vi "Indent.vi"(0 "string in":string, 1 "start indentation":i32=1) -> (2 "string out":string)   [LabVIEW 2014, in "Python Functions.lvlib"]
uses:
  Python Functions.lvlib
  <vilib>/Utility/error.llb/whitespace.ctl
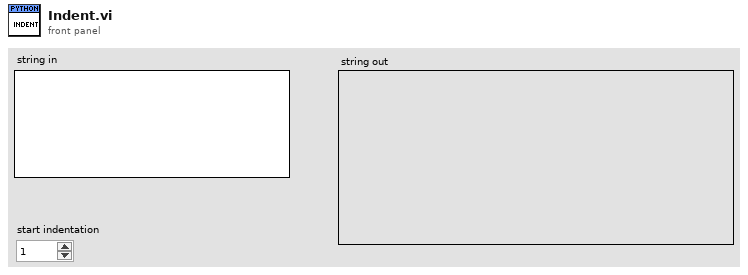
[diagram p1: front panel]
types:
  T1 = typedef "whitespace.ctl" = u16
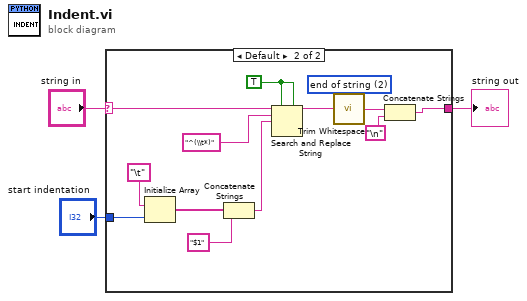
[diagram p0: block diagram]
diagram:
  n1 = case shown="Default" "string in" {
    selector: "string in" -> [_ w9]
    tunnel: [_ w5] -> w3
    tunnel: "start indentation" -> [_ w12]
    frame "" {
    }
    frame Default {
      w7 = T1 2 items=["both", "start of string", "end of string"] ("location (both)")
      w16 = TRUE ("replace all? (F)")
      n2 = Initialize Array("\t" ("String"), w12) -> (w10:string[])
      n3 = Concatenate Strings(w10, "$1" ("string")) -> (w13:string)
      n4 = Search and Replace String(replace all?=w16, multiline?=w16, input string=w9, search string="^(\\t*)", replace string=w13) -> (result string=w8:string)  [unwired: 3 in, 3 out]
      n5 = call <vilib>:"Trim Whitespace.vi"("string"=w8, "location (both)"=w7) -> ("trimmed string"=w6:string)
      n6 = Concatenate Strings(w6, "\n") -> (w5:string)
    }
  }
  "string out" <- w3
